vi "MccHat_02_Main.vi"() -> ()   [LabVIEW 2019]
uses:
  MccHat_Global.vi
panel:
  out "chart_temp 2":waveform(dbl)[](graph)=[{"t0"=timestamp(3772890114.31303 s since 1904-01-01), "dt"=1.0, "Y"=[0.8687935985565186]}, {"t0"=timestamp(3772890114.31303 s since 1904-01-01), "dt"=1.0, "Y"=[86.87935985565186]}, {"t0"=timestamp(3772890114.31303 s since 1904-01-01), "dt"=1.0, "Y"=[30.48853325313992]}, {"t0"=timestamp(3772890114.31303 s since 1904-01-01), "dt"=1.0, "Y"=[303.6385332531399]}]
  out "chart_temp":waveform(dbl)[](graph)=[{"t0"=timestamp(3772890114.31303 s since 1904-01-01), "dt"=1.0, "Y"=[0.8687935985565186]}, {"t0"=timestamp(3772890114.31303 s since 1904-01-01), "dt"=1.0, "Y"=[86.87935985565186]}, {"t0"=timestamp(3772890114.31303 s since 1904-01-01), "dt"=1.0, "Y"=[30.48853325313992]}, {"t0"=timestamp(3772890114.31303 s since 1904-01-01), "dt"=1.0, "Y"=[303.6385332531399]}]
  out "T_array":dbl[](array[numeric])
  in  "n_sample":i16=2 caption="Sample"
  in  "clear_chart":bool=TRUE caption="Clear charts to start"
  out "Last Meas. Time":timestamp format="%<%Y-%m-%d %H:%M:%S>T"
  out "name":string caption="Name"
  in  "interval":u32=2000 caption="Interval"
  out "status_init":bool caption="Initialization"
  out "status_read":bool caption="Readout"
  in  "stop":bool
  in  "port":u16=1111 caption="Port"
  in  "address":string="192.168.24.204" caption="IP Addr."
  # "MCC HAT #02"
  # "ms"
  # "per read"
  # "degC"
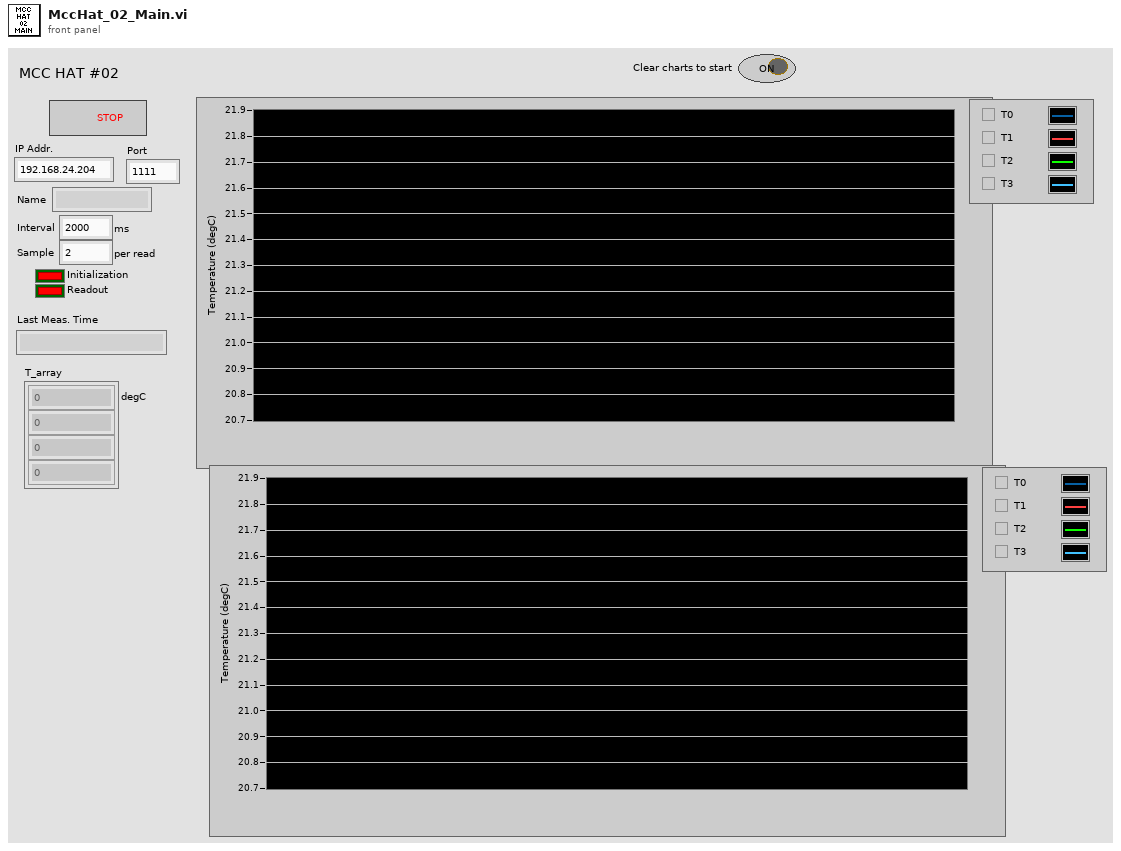
[diagram p1: front panel]
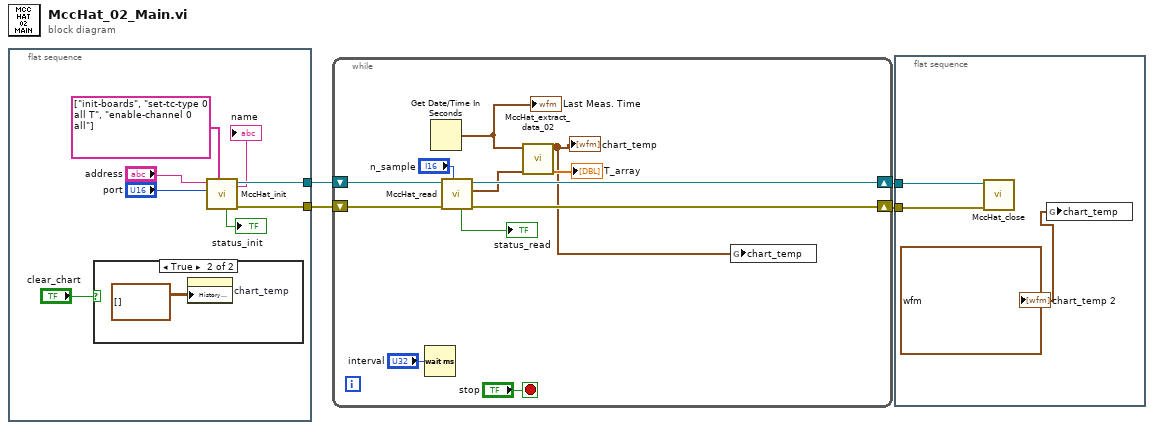
[diagram p0: block diagram]
diagram:
  n1 = flat-sequence {
    tunnel: [w10] -> w4
    tunnel: [w9] -> w3
    frame #0 {
      n2 = case shown="True" "clear_chart" {
        frame False {
        }
        frame True {
          n3 = property on="chart_temp" class="WFChart (strict)"("History Data"=waveform(dbl)[][] []) -> ()  [unwired: 2 in, 2 out]
        }
      }
      n4 = call "MccHat_init.vi"("commands"=string[] ["init-boards", "set-tc-type 0 all T", "enable-channel 0 all"], "port"="port", "address"="address") -> ("error out"=w9:errorcluster, "conn_id"=w10:refnum<k5>, "status"=→"status_init":bool, "server"=→"name":string)  [unwired: 5 in]
    }
  }
  n5 = while {
    shift-right: [w21] -> w1
    shift-left: w4 -> [w23]
    shift-right: [w20] -> w2
    shift-left: w3 -> [w22]
    stop <- "stop" stop-if-true
    n6 = Wait (ms)(milliseconds to wait="interval") -> ()  [unwired: 1 out]
    n7 = Get Date/Time In Seconds() -> (seconds since 1Jan1904=w17:timestamp)
    "Last Meas. Time" <- w17
    n8 = call "MccHat_read.vi"("n_read"="n_sample", "error in"=w22, "conn_id_in"=w23) -> ("error out"=w20:errorcluster, "readings"=w19:cluster{i32, i32, dbl}[], "conn_id_out"=w21:refnum<k5>, "status"=→"status_read":bool)  [unwired: 5 in]
    n9 = call "MccHat_extract_data_02.vi"("readings"=w19, "time"=w17) -> ("temperature_array"=→"T_array":dbl[], "waveform_array"=w14:waveform(dbl)[])  [unwired: 8 in]
    "chart_temp" <- w14
    n10 = global write "MccHat_Global.vi" "chart_temp"(w14) -> ()
  }
  n11 = flat-sequence {
    tunnel: w2 -> [w28]
    tunnel: w1 -> [w27]
    frame #0 {
      w26 = waveform(dbl)[] [{"t0"=timestamp(3789436812.8021026 s since 1904-01-01), "dt"=1.0, "Y"=[0.0]}, {"t0"=timestamp(3789436812.8021026 s since 1904-01-01), "dt"=1.0, "Y"=[21.0364]}, {"t0"=timestamp(3789436812.8021026 s since 1904-01-01), "dt"=1.0, "Y"=[20.7065]}, {"t0"=timestamp(3789436812.8021026 s since 1904-01-01), "dt"=1.0, "Y"=[-9999.0]}] ("chart_temp 2")
      n12 = call "MccHat_close.vi"("error in"=w28, "conn_id"=w27) -> ()  [unwired: 8 in, 2 out]
      n13 = global write "MccHat_Global.vi" "chart_temp"(w26) -> ()
      "chart_temp 2" <- w26
    }
  }
